vi "Test the Timer.vi"() -> ()   [LabVIEW 2012]
panel:
  out "Time done":bool
  in  "Wait Time (ms)":u32
  in  "Stop":bool
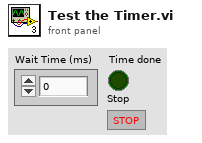
[diagram p1: front panel]
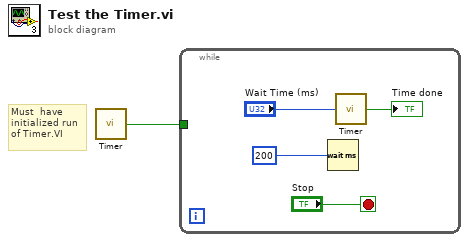
[diagram p0: block diagram]
diagram:
  # "Must  have\ninitialized run \nof Timer.VI"
  n1 = call "Timer.vi"() -> ("Time Done"=w1:bool)  [unwired: 1 in]
  n2 = while {
    tunnel: w1 -> [_]
    stop <- "Stop" stop-if-true
    n3 = Wait (ms)(milliseconds to wait=200) -> ()  [unwired: 1 out]
    n4 = call "Timer.vi"("Wait Time (ms)"="Wait Time (ms)") -> ("Time Done"=→"Time done":bool)
  }
